vi "VisualizeScope.vi"() -> ()   [LabVIEW 2018, in "Visualization.lvlib" / "VisualizeScope.lvclass"]
doc: "View data coming from the scope module based on the PluginName control."
uses:
  VisualizeScope.lvclass
  LV_Config_class/Config.lvclass/Config.ctl
  Scope/ScopeShared/ScopeData.ctl
  <vilib>/event_ctls.llb/usereventprio.ctl
  VisualizeBase/VisualizeBase_class/Requests/VisUserEventType.ctl
  Scope/ScopeShared/Waveform.ctl
  LV_Config_class/Accessors/Read Root Directory.vi
  <extravilib>/ChannelInstances/Tag-bool/Read With Abort.vi
  <extravilib>/ChannelInstances/Tag-bool/Write With Abort.vi
  <extravilib>/ChannelInstances/Tag-bool/Instantiate.vi
  <vilib>/Utility/file.llb/Write To Spreadsheet File (string).vi
  <vilib>/Utility/file.llb/Write To Spreadsheet File (DBL).vi
  <extravilib>/ChannelInstances/Tag-bool/EndpointRead.vi
  <vilib>/Utility/error.llb/Error Cluster From Error Code.vi
  <vilib>/measure/maresamp.llb/Resample Waveform (single shot).vi
  <extravilib>/ChannelInstances/Tag-bool/Endpoint.vi
  <vilib>/ErrorRing/Error Ring.xnode
  <userlib>/NIST/NISTErrorLib/NISTErrorLib.lvlib
  VisualizeBase/VisualizeBase_class/VisualizeBase.lvclass
  Scope/ScopeModule/ScopeModule.lvlib
  LV_Config_class/Config.lvclass
  <vilib>/measure/NI_MAPro.lvlib
  Scope/ScopeShared/ScopeShared.lvlib
  <extravilib>/ChannelInstances/Tag-bool.lvlib
panel:
  in  "Tab Control":T1(tab)
  out "Waveform Graph 2":waveform(dbl)[](graph)
  out "Waveform Graph":T2(graph)
  out "Waveform":waveform(dbl)[](graph)
  in  "FIR Filter Specifications":T3={"Alias Rejection (dB)"=120.0, "Normalized Bandwidth"=0.4536} {"Normalized Bandwidth" format="%.4f"; "Alias Rejection (dB)" format="%.2f"}
  out "t0 adjusted warning":bool
  in  "Interpolation Mode":u16(ring)=2 items=["coerce", "linear", "spline", "FIR filter"]
  in  "Frequency":dbl=100000000.0 format="%.2p"
  in  "btnClear":bool
  in  "btnReset":bool
  in  "btnSave":bool
  in  "btnStop":bool
  in  "PluginName":string="Scope.NIScope1"
  in  "QueName":string="ScopeVisQue"
  out "ErrorArray":errorcluster[](array[cluster])
  # "Before Filter"
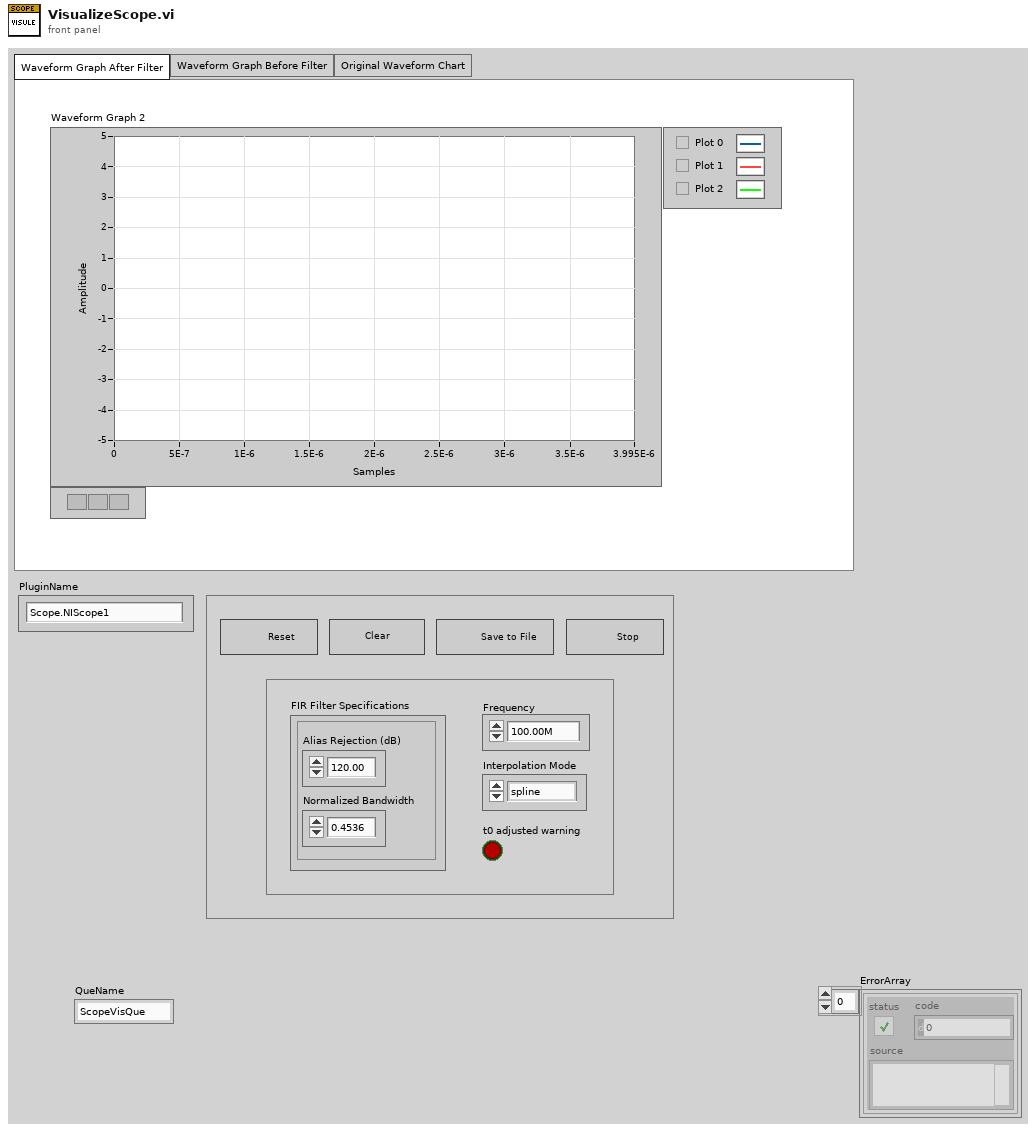
[diagram p1: front panel]
types:
  T1 = enum32{"Waveform Graph After Filter", "Waveform Graph Before Filter", "Original Waveform Chart"}
  T2 = cluster{"initial x":dbl, "x increment":dbl, "waveform array":dbl[]}[]
  T3 = cluster{"Alias Rejection (dB)":dbl, "Normalized Bandwidth":dbl}
  T4 = typedef "ScopeShared.lvlib/clBroadcastEvents.ctl" = cluster{"DidInit":refnum<user-event>, "StatusUpdate":refnum<user-event>, "ErrorReport":refnum<user-event>, "DidStop":refnum<user-event>, "PathToINI":refnum<user-event>, "Handle":refnum<user-event>, "Model":refnum<user-event>, "Channels":refnum<user-event>, "Acquisition":refnum<user-event>, "Trigger":refnum<user-event>, "ExtAcquisition":refnum<user-event>, "Waveform":refnum<user-event>}
  T5 = typedef "Visualization.lvlib/VisualizeBase.lvclass/VisRequestEvents.ctl" = cluster{"StopRequest":refnum<user-event>, "ResetRequest":refnum<user-event>, "FP Pop In or Out":refnum<user-event>}
  T6 = typedef "Visualization.lvlib/VisualizeBase.lvclass/VisUserEventType.ctl" = cluster{"BusIndex":i8, "Data":variant}
  T7 = typedef "usereventprio.ctl" = enum32{"high priority", "normal priority"}
  T8 = typedef "ScopeShared.lvlib/ScopeData.ctl" = cluster{"ScopeType":string, "ScopeData":variant}
  T9 = typedef "ScopeShared.lvlib/Waveform.ctl" = cluster{"initial x":dbl, "x increment":dbl, "waveform array":dbl[]}
  T10 = typedef "Tag-bool.lvlib/))Channel.ctl" = refnum<queue>
  T11 = typedef "Config_class.lvlib/Config.lvclass/RootDir.ctl" = cluster{"pathRootDir":path, "btnOutPath":bool, "OutDir":string, "btnOpenOutputDir":bool, "ScriptDir":string, "btnOpenScriptDir":bool, "TestDir":string, "btnOpenTestDir":bool}
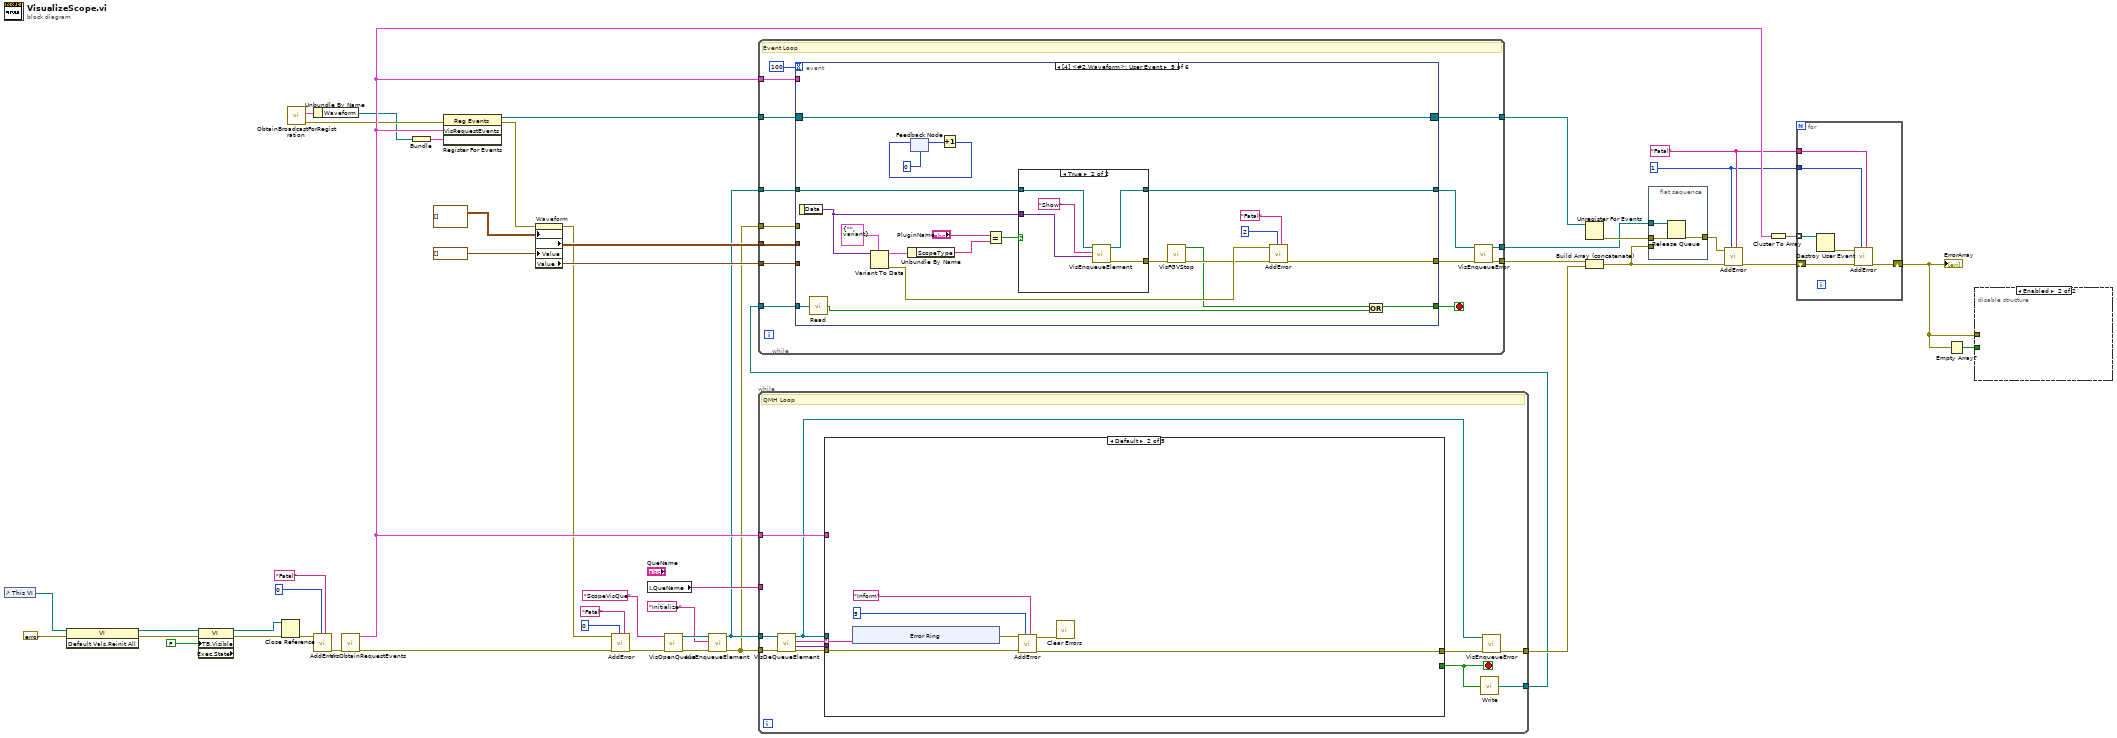
[diagram p0: block diagram]
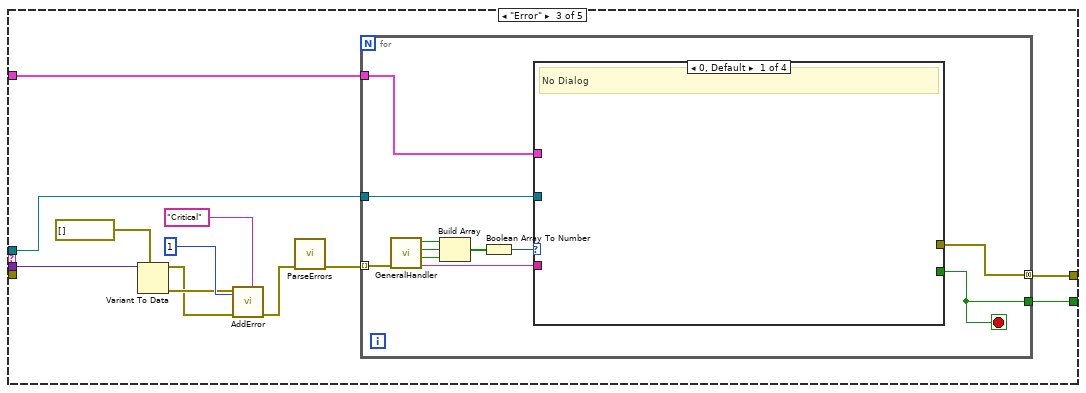
[diagram p3: hidden frame]
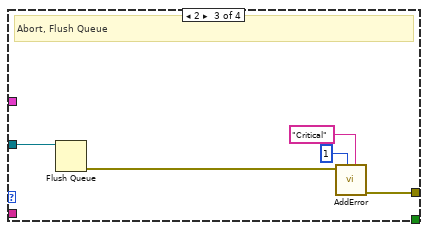
[diagram p5: hidden frame]
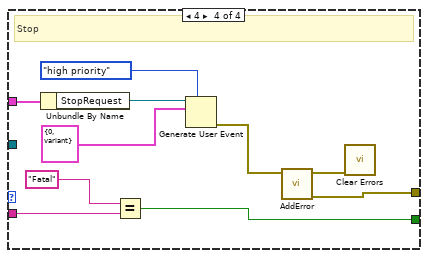
[diagram p6: hidden frame]
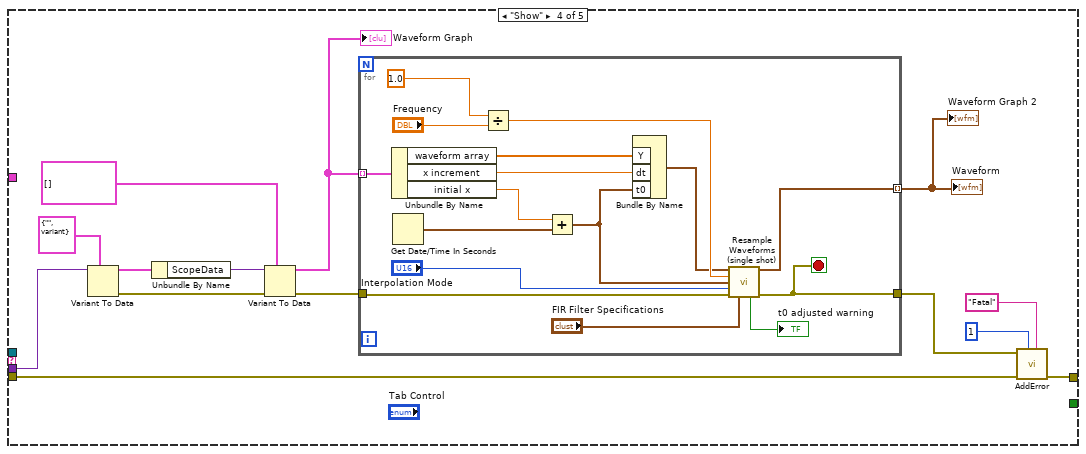
[diagram p7: hidden frame]
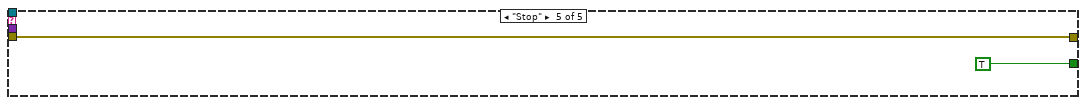
[diagram p8: hidden frame]
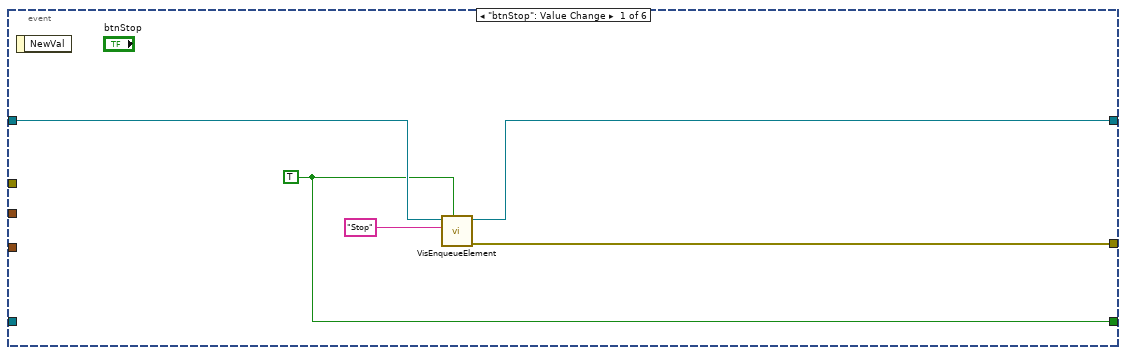
[diagram p9: hidden frame]
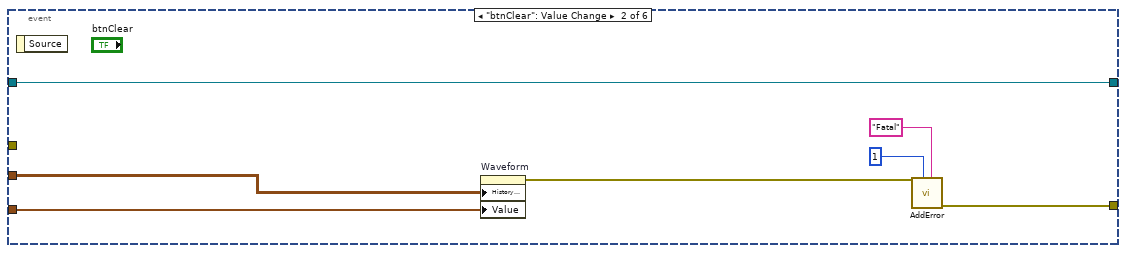
[diagram p10: hidden frame]
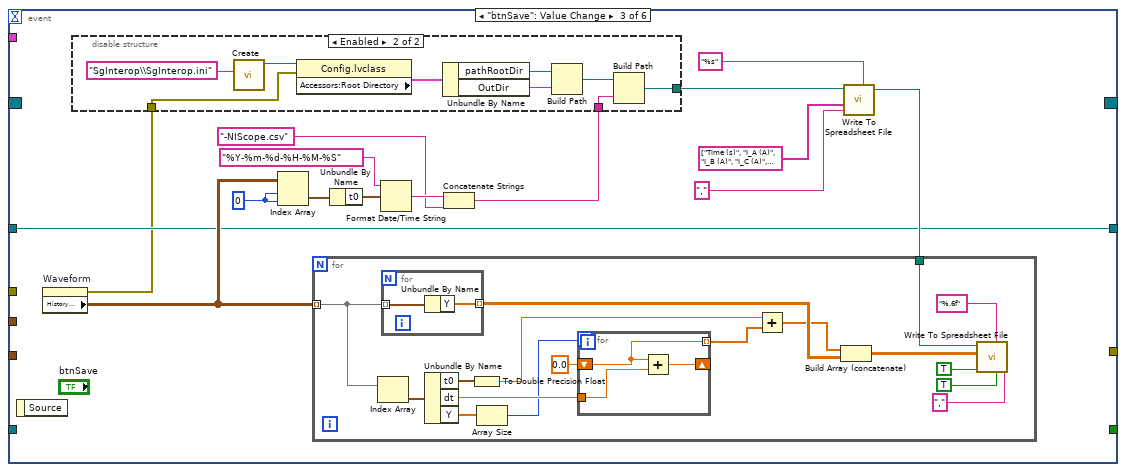
[diagram p11: hidden frame]
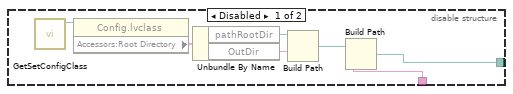
[diagram p12: hidden frame]
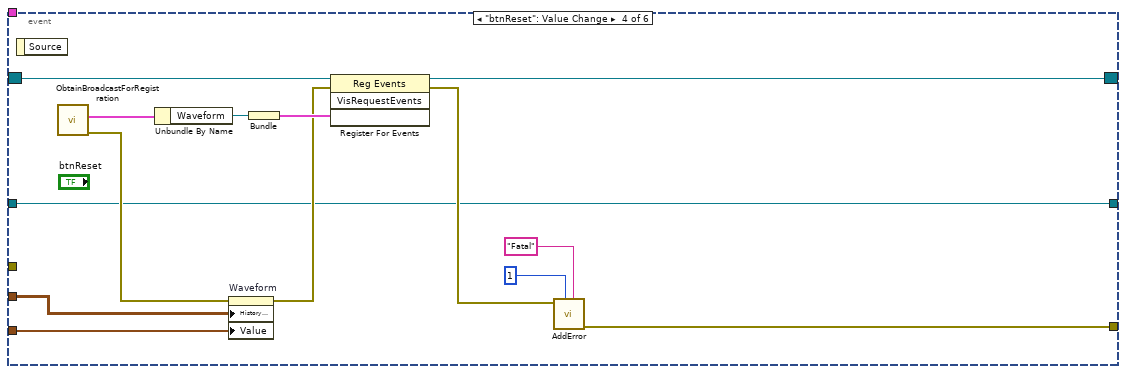
[diagram p13: hidden frame]
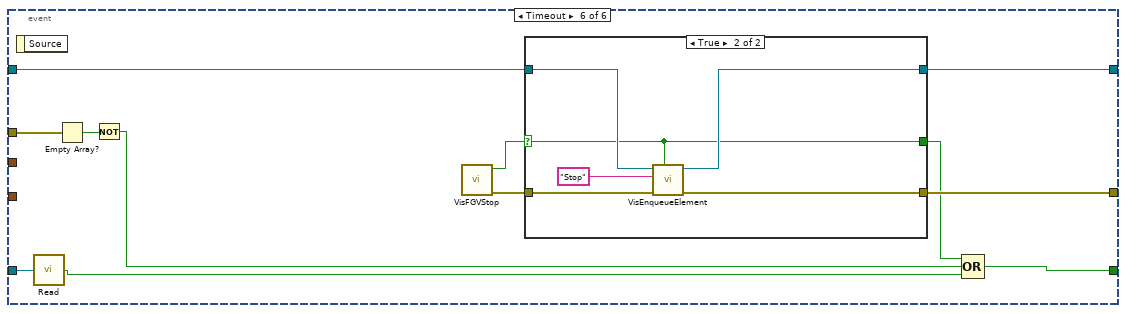
[diagram p15: hidden frame]
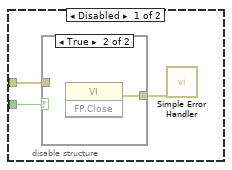
[diagram p17: hidden frame]
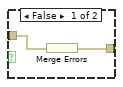
[diagram p18: hidden frame]
diagram:
  w8 = "Fatal" ("Severity")
  w7 = u8 1 ("Priority")
  n1 = control-ref of="This VI"() -> (w25:refnum<vi>)
  n2 = invoke class="VI" method="Default Vals.Reinit All"(reference=w25, error in=errorcluster {"status"=FALSE, "code"=0, "source"=""} ("error in (no error)")) -> (reference out=w4:refnum<vi>, error out=w5:errorcluster)  [unwired: 1 in, 1 out]
  n3 = property class="VI" props=["TB.Visible", "Exec.State"](reference=w4, error in=w5, "TB.Visible"=FALSE ("Tool Bar:Show Run Button")) -> (reference out=w3:refnum<vi>, error out=w2:errorcluster)  [unwired: 1 out]
  n4 = Close Reference(reference=w3, error in (no error)=w2) -> (error out=w23:errorcluster)
  n5 = call "ObtainBroadcastForRegistration.vi"() -> ("error out"=w37:errorcluster, "ScopeBroadcastEvents"=w36:T4)  [unwired: 10 in]
  n6 = Unbundle By Name(w36) -> ("Waveform"=w35:refnum<user-event>)
  n7 = call <userlib>:"AddError.vi"("Severity"="Fatal", "Priority"=u8 0, "error in (no error)"=w23) -> ("ErrorArray Out"=w47:errorcluster[])  [unwired: 7 in, 1 out]
  n8 = call "VisObtainRequestEvents.vi"("Error"=w47) -> ("Error"=w18:errorcluster[], "VisRequestEvents"=w38:T5)  [unwired: 9 in]
  n9 = Bundle("Waveform"=w35) -> (w34:cluster{"Waveform":refnum<user-event>})  [unwired: 1 in]
  n10 = register-events(error in=w37, w38, w34) -> (reference out=w48:refnum<event-registration>, error out=w33:errorcluster)  [unwired: 1 in]
  n11 = property on="Waveform" class="WFChart (strict)"(error in=w33, "History Data"=waveform(dbl)[][] [], "Value"=waveform(dbl)[] [] ("Waveform")) -> (error out=w17:errorcluster, "History Data"=w27:waveform(dbl)[][], "Value"=w28:waveform(dbl)[])  [unwired: 1 in, 1 out]
  n12 = call <userlib>:"AddError.vi"("Severity"="Fatal", "Priority"=u8 0, "ErrorArray In"=w18, "error in (no error)"=w17) -> ("ErrorArray Out"=w13:errorcluster[])  [unwired: 6 in, 1 out]
  n13 = local read "QueName"() -> (w46:string)
  n14 = call "VisOpenQueue.vi"("Error Array In"=w13, "QueueName"="ScopeVisQue" ("QueName 2")) -> ("Error Array Out"=w16:errorcluster[], "queue out"=w15:refnum<queue>)  [unwired: 8 in]
  n15 = call "VisEnqueueElement.vi"("Error Array In"=w16, "Message"="Initialize", "queue in"=w15) -> ("Error Array Out"=w6:errorcluster[], "queue out"=w11:refnum<queue>)  [unwired: 7 in]
  n16 = while {
    tunnel: w6 -> [w56]
    tunnel: [w50] -> w42
    tunnel: w46 -> [_]
    tunnel: w38 -> [w58]
    tunnel: [w57] -> w30
    tunnel: w11 -> [w52]
    stop <- w59 stop-if-true
    # "QMH Loop"
    n17 = call "VisDeQueueElement.vi"("Error Array In"=w56, "Queue In"=w52) -> ("Error Array Out"=w54:errorcluster[], "Data"=w53:variant, "Message"=w55:string, "Queue Out"=w49:refnum<queue>)  [unwired: 6 in]
    n18 = case shown="Default" w55 {
      selector: w55 -> [_ w67 _ _ _]
      tunnel: w53 -> [_ _ w86 w118 _]
      tunnel: w54 -> [w60 w65 _ w114 w143]
      tunnel: [w60 w64 w83 w126 w143] -> w51
      tunnel: [_ _ w82 _ TRUE] -> w59
      tunnel: w58 -> [_ _ w81 _ _]
      tunnel: w49 -> [_ _ w75 _ _]
      frame "Initialize" {
      }
      frame Default {
        n19 = xnode "Error Ring"("parameter 0"=w67) -> ("error out"=w66:errorcluster)
        n20 = call <userlib>:"AddError.vi"("Severity"="Inform" ("String"), "Priority"=u8 5, "ErrorArray In"=w65, "error in (no error)"=w66) -> ("ErrorArray Out"=w64:errorcluster[], "error out"=w63:errorcluster)  [unwired: 6 in]
        n21 = call <vilib>:"Clear Errors.vi"("error in (no error)"=w63) -> ()  [unwired: 5 in, 2 out]
      }
      frame "Error" {
        n22 = Variant To Data(type=errorcluster[] [], Variant=w86) -> (data=w77:errorcluster[], error out=w78:errorcluster)  [unwired: 1 in]
        n23 = call <userlib>:"AddError.vi"("Severity"="Critical" ("String"), "Priority"=u8 1, "ErrorArray In"=w77, "error in (no error)"=w78) -> ("ErrorArray Out"=w76:errorcluster[])  [unwired: 6 in, 1 out]
        n24 = call <userlib>:"ParseErrors.vi"("ErrorArray"=w76) -> ("ErrorArray"=w84:errorcluster[])  [unwired: 8 in, 2 out]
        n25 = for {
          tunnel: w84 -> [w97] mode=indexing
          tunnel: [w91] -> w83 mode=concatenating
          tunnel: [w89] -> w82
          tunnel: w81 -> [w88]
          tunnel: w75 -> [w87]
          stop <- w89 stop-if-true
          n26 = call <userlib>:"GeneralHandler.vi"("error in (no error)"=w97) -> ("Severity"=w90:string, "Stop"=w94:bool, "Abort"=w95:bool, "Continue"=w96:bool)  [unwired: 6 in, 1 out]
          n27 = Build Array(w96, w95, w94) -> (w93:bool[])
          n28 = Boolean Array To Number(Boolean array=w93) -> (number=w92:u32)
          n29 = case shown="0, Default" w92 {
            tunnel: [_ _ w102 w111] -> w91
            tunnel: w90 -> [_ _ _ w106]
            tunnel: [_ _ _ w104] -> w89
            tunnel: w88 -> [_ _ _ w103]
            tunnel: w87 -> [_ _ w98 _]
            frame 0, Default {
              # "No Dialog"
            }
            frame 1 {
              # "Continue"
            }
            frame 2 {
              # "Abort, Flush Queue"
              n30 = Flush Queue(queue=w98) -> (error out=w101:errorcluster)  [unwired: 1 in, 2 out]
              n31 = call <userlib>:"AddError.vi"("Severity"="Critical" ("String"), "Priority"=u8 1, "error in (no error)"=w101) -> ("ErrorArray Out"=w102:errorcluster[])  [unwired: 7 in, 1 out]
            }
            frame 4 {
              # "Stop"
              n32 = Unbundle By Name(w103) -> ("StopRequest"=w112:refnum<user-event>)
              n33 = Equal?(x="Fatal", y=w106) -> (x = y?=w104:bool)
              n34 = Generate User Event(priority (normal)=usereventprio."high priority", user event=w112, event data cluster=T6 {"BusIndex"=0, "Data"=variant} ("event data")) -> (error out=w110:errorcluster)  [unwired: 1 in, 1 out]
              n35 = call <userlib>:"AddError.vi"("error in (no error)"=w110) -> ("ErrorArray Out"=w111:errorcluster[], "error out"=w107:errorcluster)  [unwired: 9 in]
              n36 = call <vilib>:"Clear Errors.vi"("error in (no error)"=w107) -> ()  [unwired: 5 in, 2 out]
            }
          }
        }
      }
      frame "Show" {
        n37 = Variant To Data(type=T8 {"ScopeType"="", "ScopeData"=variant} ("ScopeData"), Variant=w118) -> (data=w120:T8, error out=w116:errorcluster)  [unwired: 1 in]
        n38 = Unbundle By Name(w120) -> ("ScopeData"=w117:variant)
        n39 = Variant To Data(error in=w116, type=T9[] [], Variant=w117) -> (data=w115:T9[], error out=w122:errorcluster)
        "Waveform Graph" <- w115
        n40 = for {
          tunnel: w115 -> [w142] mode=indexing
          tunnel: [w141] -> w113 mode=indexing
          tunnel: [w133] -> w123
          tunnel: w122 -> [w127]
          stop <- w133 stop-if-true
          n41 = Unbundle By Name(w142) -> ("waveform array"=w140:dbl[], "x increment"=w139:dbl, "initial x"=w129:dbl)
          n42 = Get Date/Time In Seconds() -> (seconds since 1Jan1904=w130:timestamp)
          n43 = Divide(x=1.0, y="Frequency") -> (x/y=w134:dbl)
          n44 = Add(x=w129, y=w130) -> (x+y=w128:timestamp)
          n45 = Bundle By Name("Y"=w140, "dt"=w139, "t0"=w128) -> (w132:waveform(dbl))  [unwired: 1 in]
          n46 = call-poly <vilib>:"Resample Waveforms (single shot).vi"("waveform in"=w132, "dt"=w134, "t0"=w128, "interpolation mode"="Interpolation Mode", "error in (no error)"=w127, "FIR filter specifications"="FIR Filter Specifications") -> ("resampled waveform out"=w141:waveform(dbl), "t0 adjusted warning"=→"t0 adjusted warning":bool, "error out"=w133:errorcluster)  [unwired: 6 in, 1 out]
        }
        "Waveform" <- w113
        "Waveform Graph 2" <- w113
        n47 = call <userlib>:"AddError.vi"("Severity"="Fatal", "Priority"=u8 1, "ErrorArray In"=w114, "error in (no error)"=w123) -> ("ErrorArray Out"=w126:errorcluster[])  [unwired: 6 in, 1 out]
      }
      frame "Stop" {
      }
    }
    n48 = call <extravilib>:"Write.vi"("element"=w59) -> ("channel"=w57:T10)  [unwired: 1 out]
    n49 = call "VisEnqueueError.vi"("Error Array In"=w51, "Queue in"=w49) -> ("Error Array Out"=w50:errorcluster[])  [unwired: 8 in, 1 out]
  }
  n50 = while {
    tunnel: w48 -> [w158]
    tunnel: [w146] -> w43
    tunnel: [w156] -> w45
    tunnel: w38 -> [w155]
    tunnel: w6 -> [w154]
    tunnel: w28 -> [w153]
    tunnel: w27 -> [w152]
    tunnel: w30 -> [w150]
    tunnel: w11 -> [w149]
    tunnel: [w145] -> w10
    stop <- w157 stop-if-true
    # "Event Loop"
    n51 = event shown="[4] <#2.Waveform>: User Event" {
      selector: w158 -> [_ _ _ w236 w248 _]
      dyn-events: [_ _ _ w235 w248 _] -> w156
      timeout: 100 -> [_ _ _ _ _ _]
      tunnel: [w161 _ _ _ w243 w273] -> w157
      tunnel: [w160 w170 _ w237 w257 w270] -> w147
      tunnel: w155 -> [_ _ _ _ _ _]
      tunnel: w154 -> [_ _ _ _ _ w269]
      tunnel: w153 -> [_ w167 _ w230 _ _]
      tunnel: w152 -> [_ w168 _ w229 _ _]
      tunnel: w150 -> [_ _ _ _ w259 w277]
      tunnel: [w159 w166 w172 w226 w249 w271] -> w148
      tunnel: w149 -> [w162 w166 w172 w226 w252 w274]
      event "btnStop": Value Change {
        w161 = TRUE ("Priority? (F)")
        n52 = event-data() -> ()  [unwired: 1 in, 1 out]
        n53 = call "VisEnqueueElement.vi"("Priority? (F)"=w161, "Message"="Stop", "queue in"=w162) -> ("Error Array Out"=w160:errorcluster[], "queue out"=w159:refnum<queue>)  [unwired: 7 in]
      }
      event "btnClear": Value Change {
        n54 = event-data() -> ()  [unwired: 1 in, 1 out]
        n55 = property on="Waveform" class="WFChart (strict)"("History Data"=w168, "Value"=w167) -> (error out=w169:errorcluster)  [unwired: 2 in, 1 out]
        n56 = call <userlib>:"AddError.vi"("Severity"="Fatal", "Priority"=u8 1, "error in (no error)"=w169) -> ("ErrorArray Out"=w170:errorcluster[])  [unwired: 7 in, 1 out]
      }
      event "btnSave": Value Change {
        w175 = 0 ("index (row)")
        n57 = event-data() -> ()  [unwired: 1 in, 1 out]
        n58 = property on="Waveform" class="WFChart (strict)"() -> (error out=w171:errorcluster, "History Data"=w176:waveform(dbl)[][])  [unwired: 2 in, 1 out]
        n59 = Index Array(array=w176, index (row)=w175, index (col)=w175) -> (element=w174:waveform(dbl))
        n60 = Unbundle By Name(w174) -> ("t0"=w173:timestamp)
        n61 = Format Date/Time String(time format string (%c)="%Y-%m-%d-%H-%M-%S", seconds (now)=w173) -> (date/time string=w184:string)  [unwired: 1 in]
        n62 = Concatenate Strings(w184, "-NIScope.csv" ("string")) -> (w182:string)
        n63 = disable-structure shown="Enabled" {
          disable-tunnel: [w214 w216] -> w181
          disable-tunnel: w182 -> [w208 w217]
          disable-tunnel: w171 -> [_ w215]
          frame Disabled {
            n64 = call "GetSetConfigClass.vi"() -> ("Ref out"=w212:refnum<class "Config.lvclass">)  [unwired: 11 in]
            n65 = property class="Config.lvclass"(reference=w212) -> ("Accessors:Root Directory"=w211:T11)  [unwired: 1 in, 2 out]
            n66 = Unbundle By Name(w211) -> ("pathRootDir"=w210:path, "OutDir"=w209:string)
            n67 = Build Path(base path=w210, name or relative path=w209) -> (appended path=w213:path)
            n68 = Build Path(base path=w213, name or relative path=w208) -> (appended path=w214:path)
          }
          frame Enabled {
            n69 = call "Create.vi"("name or relative path"="SgInterop\\SgInterop.ini") -> ("Ref out"=w222:refnum<class "Config.lvclass">)  [unwired: 9 in, 1 out]
            n70 = property class="Config.lvclass"(reference=w222, error in=w215) -> ("Accessors:Root Directory"=w221:T11)  [unwired: 2 out]
            n71 = Unbundle By Name(w221) -> ("pathRootDir"=w220:path, "OutDir"=w219:string)
            n72 = Build Path(base path=w220, name or relative path=w219) -> (appended path=w218:path)
            n73 = Build Path(base path=w218, name or relative path=w217) -> (appended path=w216:path)
          }
        }
        n74 = call-poly <vilib>:"Write To Spreadsheet File.vi"("delimiter (\\t)"="," ("delimiter (\\t)"), "format (%s)"="%s" ("format (%.3f)"), "1D data"=string[] ["Time (s)", "I_A (A)", "I_B (A)", "I_C (A)", "V_A (V)", "V_B (V)", "V_C (V)"], "file path (dialog if empty)"=w181) -> ("new file path (Not A Path if cancelled)"=w180:path)  [unwired: 4 in]
        n75 = for {
          tunnel: w180 -> [w197]
          tunnel: w176 -> [w191] mode=indexing
          n76 = Index Array(array=w191) -> (element=w190:waveform(dbl))  [unwired: 1 in]
          n77 = for {
            tunnel: w191 -> [w207] mode=indexing
            tunnel: [w206] -> w196 mode=indexing
            n78 = Unbundle By Name(w207) -> ("Y"=w206:dbl[])
          }
          n79 = Unbundle By Name(w190) -> ("t0"=w195:timestamp, "dt"=w194:dbl, "Y"=w193:dbl[])
          n80 = To Double Precision Float(number=w195) -> (double precision float=w187:dbl)
          n81 = Array Size(array=w193) -> (size(s)=w192:i32)
          n82 = for {
            N: w192 -> [_]
            tunnel: w194 -> [w205]
            shift-right: [w204] -> _
            shift-left: 0.0 -> [w203]
            tunnel: [w203] -> w188 mode=indexing
            n83 = Add(x=w203, y=w205) -> (x+y=w204:dbl)
          }
          n84 = Add(x=w187, y=w188) -> (x+y=w186:dbl[])
          n85 = Build Array (concatenate)(w186, w196) -> (w202:dbl[][])
          n86 = call-poly <vilib>:"Write To Spreadsheet File.vi"("delimiter (\\t)"="," ("delimiter (\\t)"), "transpose? (no:F)"=TRUE, "format (%.3f)"="%.6f", "append to file? (new file:F)"=TRUE, "2D data"=w202, "file path (dialog if empty)"=w197) -> ()  [unwired: 2 in, 1 out]
        }
      }
      event "btnReset": Value Change {
        n87 = event-data() -> ()  [unwired: 1 in, 1 out]
        n88 = call "ObtainBroadcastForRegistration.vi"() -> ("error out"=w231:errorcluster, "ScopeBroadcastEvents"=w232:T4)  [unwired: 10 in]
        n89 = Unbundle By Name(w232) -> ("Waveform"=w234:refnum<user-event>)
        n90 = property on="Waveform" class="WFChart (strict)"(error in=w231, "History Data"=w229, "Value"=w230) -> (error out=w228:errorcluster)  [unwired: 1 in, 1 out]
        n91 = Bundle("Waveform"=w234) -> (w233:cluster{"Waveform":refnum<user-event>})  [unwired: 1 in]
        n92 = register-events(reference=w236, error in=w228, w233) -> (reference out=w235:refnum<event-registration>, error out=w227:errorcluster)  [unwired: 1 in]
        n93 = call <userlib>:"AddError.vi"("Severity"="Fatal", "Priority"=u8 1, "error in (no error)"=w227) -> ("ErrorArray Out"=w237:errorcluster[])  [unwired: 7 in, 1 out]
      }
      event User Event {
        n94 = event-data() -> ("Data"=w253:variant)  [unwired: 1 in]
        n95 = call <extravilib>:"Read.vi"("channel"=w259) -> ("element"=w242:bool)  [unwired: 1 in, 1 out]
        n96 = Variant To Data(type=T8 {"ScopeType"="", "ScopeData"=variant} ("ScopeData"), Variant=w253) -> (data=w256:T8, error out=w241:errorcluster)  [unwired: 1 in]
        n97 = Unbundle By Name(w256) -> ("ScopeType"=w255:string)
        n98 = feedback #1(0) -> (w247:i32)
        n99 = Increment(x=w247) -> (x+1=w245:i32)
        n100 = feedback-in #1(w245) -> ()
        n101 = Equal?(x="PluginName", y=w255) -> (x = y?=w251:bool)
        n102 = case shown="True" w251 {
          tunnel: [_ w265] -> w240
          tunnel: w252 -> [w260 w264]
          tunnel: [w260 w262] -> w249
          tunnel: w253 -> [_ w263]
          frame False {
          }
          frame True {
            n103 = call "VisEnqueueElement.vi"("Data"=w263, "Message"="Show", "queue in"=w264) -> ("Error Array Out"=w265:errorcluster[], "queue out"=w262:refnum<queue>)  [unwired: 7 in]
          }
        }
        n104 = call "VisFGVStop.vi"("Error In"=w240) -> ("Error Out"=w239:errorcluster[], "Value"=w238:bool)  [unwired: 9 in]
        n105 = call <userlib>:"AddError.vi"("Severity"="Fatal", "Priority"=u8 2, "ErrorArray In"=w239, "error in (no error)"=w241) -> ("ErrorArray Out"=w257:errorcluster[])  [unwired: 6 in, 1 out]
        n106 = Or(x=w238, y=w242) -> (x .or. y?=w243:bool)
      }
      event Timeout {
        n107 = event-data() -> ()  [unwired: 1 in, 1 out]
        n108 = call <extravilib>:"Read.vi"("channel"=w277) -> ("element"=w272:bool)  [unwired: 1 in, 1 out]
        n109 = Empty Array?(array=w269) -> (empty?=w268:bool)
        n110 = Not(x=w268) -> (.not. x?=w266:bool)
        n111 = call "VisFGVStop.vi"() -> ("Error Out"=w275:errorcluster[], "Value"=w276:bool)  [unwired: 10 in]
        n112 = case shown="True" w276 {
          selector: w276 -> [w278 w281]
          tunnel: [w280 w284] -> w270
          tunnel: w275 -> [w280 w285]
          tunnel: w274 -> [w279 w283]
          tunnel: [w279 w282] -> w271
          tunnel: [w278 w281] -> w267
          frame False {
          }
          frame True {
            n113 = call "VisEnqueueElement.vi"("Priority? (F)"=w281, "Error Array In"=w285, "Message"="Stop", "queue in"=w283) -> ("Error Array Out"=w284:errorcluster[], "queue out"=w282:refnum<queue>)  [unwired: 6 in]
          }
        }
        n114 = Compound Arithmetic op=OR(w267, w266, w272) -> (w273:bool)
      }
    }
    n115 = call "VisEnqueueError.vi"("Error Array In"=w147, "Queue in"=w148) -> ("Error Array Out"=w146:errorcluster[], "Queue out"=w145:refnum<queue>)  [unwired: 8 in]
  }
  n116 = Unregister For Events(event registration refnum=w45) -> (error out=w41:errorcluster)  [unwired: 1 in]
  n117 = Build Array (concatenate)(w43, w42) -> (w9:errorcluster[])
  n118 = flat-sequence {
    tunnel: w41 -> [w289]
    tunnel: [w288] -> w40
    tunnel: w10 -> [w287]
    tunnel: w9 -> [_]
    frame #0 {
      n119 = Release Queue(queue=w287, error in (no error)=w289) -> (error out=w288:errorcluster)  [unwired: 1 in, 2 out]
    }
  }
  n120 = call <userlib>:"AddError.vi"("Severity"=w8, "Priority"=w7, "ErrorArray In"=w9, "error in (no error)"=w40) -> ("ErrorArray Out"=w39:errorcluster[])  [unwired: 6 in, 1 out]
  n121 = Cluster To Array(cluster=w38) -> (array=w44:refnum<user-event>[])
  n122 = for {
    tunnel: w44 -> [w295] mode=indexing
    shift-right: [w294] -> w26
    shift-left: w39 -> [w293]
    tunnel: w8 -> [w291]
    tunnel: w7 -> [w290]
    n123 = Destroy User Event(user event=w295) -> (error out=w292:errorcluster)  [unwired: 1 in]
    n124 = call <userlib>:"AddError.vi"("Severity"=w291, "Priority"=w290, "ErrorArray In"=w293, "error in (no error)"=w292) -> ("ErrorArray Out"=w294:errorcluster[])  [unwired: 6 in, 1 out]
  }
  "ErrorArray" <- w26
  n125 = Empty Array?(array=w26) -> (empty?=w32:bool)
  n126 = disable-structure shown="Enabled" {
    disable-tunnel: w32 -> [w298 _]
    disable-tunnel: w26 -> [w296 _]
    frame Disabled {
      n127 = case shown="True" w298 {
        tunnel: [w300 w301] -> w297
        tunnel: w296 -> [w299 _]
        frame False {
          n128 = Merge Errors(w299) -> (w300:errorcluster)
        }
        frame True {
          n129 = invoke class="VI" method="FP.Close"() -> (error out=w301:errorcluster)  [unwired: 3 in, 2 out]
        }
      }
      n130 = call <vilib>:"Simple Error Handler.vi"("error in (no error)"=w297) -> ()  [unwired: 4 in, 5 out]
    }
    frame Enabled {
    }
  }
